vi "UpdateLibraryFromTemplate.vi"(8 "error in (no error)":errorcluster, 10 "Prototype Library Path":path, 11 "Target Library":refnum<vi>) -> (0 "error out":errorcluster, 3 "Target Library Out":refnum<vi>)   [LabVIEW 2019, in "gRPC Template Creation Utility.lvlib"]
uses:
  gRPC Template Creation Utility.lvlib
  <vilib>/LabVIEW Icon API/LabVIEW Icon API.lvlib
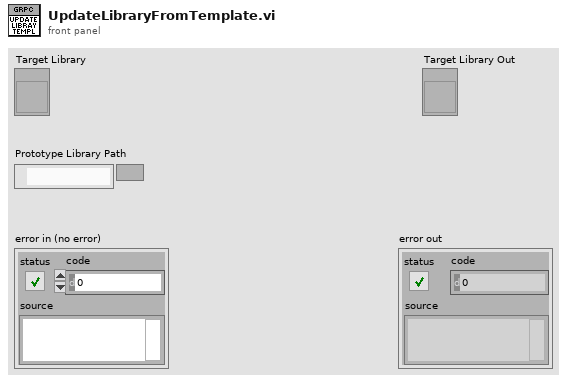
[diagram p1: front panel]
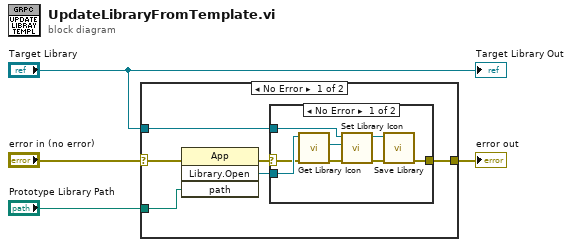
[diagram p0: block diagram]
diagram:
  n1 = case shown="No Error" "error in (no error)" {
    selector: "error in (no error)" -> [w7 w20]
    tunnel: "Target Library" -> [w8 _]
    tunnel: [w6 w20] -> w2
    tunnel: "Prototype Library Path" -> [w5 _]
    frame No Error {
      n2 = invoke class="App" method="Library.Open"(error in=w7, "path"=w5) -> (error out=w10:errorcluster, "Open Library"=w9:refnum<vi>)  [unwired: 2 in, 2 out]
      n3 = case shown="No Error" w10 {
        selector: w10 -> [w12 w19]
        tunnel: w9 -> [w18 _]
        tunnel: w8 -> [w16 _]
        tunnel: [w11 w19] -> w6
        frame No Error {
          n4 = call <vilib>:"Get Library Icon.vi"("error in (no error)"=w12, "Library Refnum in"=w18) -> ("error out"=w13:errorcluster, "Icon"=w17:refnum<class "Icon.lvclass">)  [unwired: 7 in, 1 out]
          n5 = call <vilib>:"Set Library Icon.vi"("error in (no error)"=w13, "Icon"=w17, "Library Refnum in"=w16) -> ("error out"=w14:errorcluster, "Library Refnum out"=w15:refnum<vi>)  [unwired: 7 in]
          n6 = call "Save Library.vi"("error in (no error)"=w14, "Library in"=w15) -> ("error out"=w11:errorcluster)  [unwired: 8 in, 1 out]
        }
        frame Error {
        }
      }
    }
    frame Error {
    }
  }
  "error out" <- w2
  "Target Library Out" <- "Target Library"
